vi "DDPoseEst2_Traj_DashWrite.vi"   [LabVIEW 2019]
uses:
  DDPoseEst2_Traj_Globals.vi
  <vilib>/Rock Robotics/Network Tables/NT Write Number.vi
  <vilib>/Rock Robotics/Network Tables/NT Write Boolean.vi
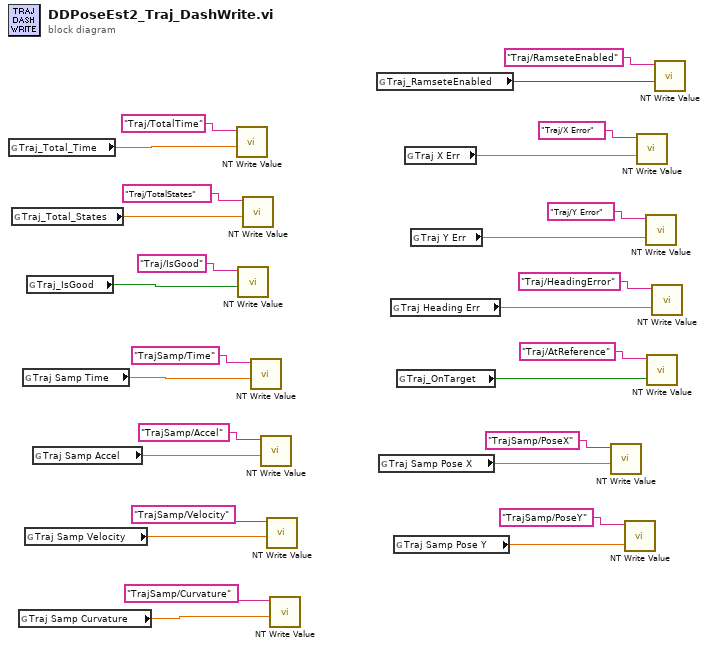
[diagram p0: block diagram]
diagram:
  n1 = global read "DDPoseEst2_Traj_Globals.vi" "Traj_Total_Time"() -> (w14:dbl)
  n2 = global read "DDPoseEst2_Traj_Globals.vi" "Traj_Total_States"() -> (w13:dbl)
  n3 = global read "DDPoseEst2_Traj_Globals.vi" "Traj Samp Curvature"() -> (w8:dbl)
  n4 = global read "DDPoseEst2_Traj_Globals.vi" "Traj Samp Time"() -> (w11:dbl)
  n5 = global read "DDPoseEst2_Traj_Globals.vi" "Traj Samp Velocity"() -> (w9:dbl)
  n6 = global read "DDPoseEst2_Traj_Globals.vi" "Traj_IsGood"() -> (w12:bool)
  n7 = global read "DDPoseEst2_Traj_Globals.vi" "Traj Samp Accel"() -> (w10:dbl)
  n8 = call-poly <vilib>:"NT Write Value.vi"("value"=w14, "name"="Traj/TotalTime" ("Name")) -> ()  [unwired: 9 in, 1 out]
  n9 = call-poly <vilib>:"NT Write Value.vi"("value"=w12, "name"="Traj/IsGood" ("Name")) -> ()  [unwired: 9 in, 1 out]
  n10 = call-poly <vilib>:"NT Write Value.vi"("value"=w13, "name"="Traj/TotalStates" ("Name")) -> ()  [unwired: 9 in, 1 out]
  n11 = call-poly <vilib>:"NT Write Value.vi"("value"=w11, "name"="TrajSamp/Time" ("Name")) -> ()  [unwired: 9 in, 1 out]
  n12 = call-poly <vilib>:"NT Write Value.vi"("value"=w10, "name"="TrajSamp/Accel" ("Name")) -> ()  [unwired: 9 in, 1 out]
  n13 = call-poly <vilib>:"NT Write Value.vi"("value"=w9, "name"="TrajSamp/Velocity" ("Name")) -> ()  [unwired: 9 in, 1 out]
  n14 = call-poly <vilib>:"NT Write Value.vi"("value"=w8, "name"="TrajSamp/Curvature" ("Name")) -> ()  [unwired: 9 in, 1 out]
  n15 = global read "DDPoseEst2_Traj_Globals.vi" "Traj_RamseteEnabled"() -> (w7:bool)
  n16 = global read "DDPoseEst2_Traj_Globals.vi" "Traj Samp Pose X"() -> (w2:dbl)
  n17 = global read "DDPoseEst2_Traj_Globals.vi" "Traj Heading Err"() -> (w4:dbl)
  n18 = global read "DDPoseEst2_Traj_Globals.vi" "Traj Samp Pose Y"() -> (w1:dbl)
  n19 = global read "DDPoseEst2_Traj_Globals.vi" "Traj_OnTarget"() -> (w3:bool)
  n20 = global read "DDPoseEst2_Traj_Globals.vi" "Traj X Err"() -> (w6:dbl)
  n21 = global read "DDPoseEst2_Traj_Globals.vi" "Traj Y Err"() -> (w5:dbl)
  n22 = call-poly <vilib>:"NT Write Value.vi"("value"=w2, "name"="TrajSamp/PoseX" ("Name")) -> ()  [unwired: 9 in, 1 out]
  n23 = call-poly <vilib>:"NT Write Value.vi"("value"=w1, "name"="TrajSamp/PoseY" ("Name")) -> ()  [unwired: 9 in, 1 out]
  n24 = call-poly <vilib>:"NT Write Value.vi"("value"=w6, "name"="Traj/X Error" ("Name")) -> ()  [unwired: 9 in, 1 out]
  n25 = call-poly <vilib>:"NT Write Value.vi"("value"=w5, "name"="Traj/Y Error" ("Name")) -> ()  [unwired: 9 in, 1 out]
  n26 = call-poly <vilib>:"NT Write Value.vi"("value"=w3, "name"="Traj/AtReference" ("Name")) -> ()  [unwired: 9 in, 1 out]
  n27 = call-poly <vilib>:"NT Write Value.vi"("value"=w4, "name"="Traj/HeadingError" ("Name")) -> ()  [unwired: 9 in, 1 out]
  n28 = call-poly <vilib>:"NT Write Value.vi"("value"=w7, "name"="Traj/RamseteEnabled" ("Name")) -> ()  [unwired: 9 in, 1 out]
